vi "AIT 1553 Channel Page.vi"(8 "error in (no error)":errorcluster, 11 "Node Ptr":T1 format="%.0x") -> (0 "error out":errorcluster)   [LabVIEW 2013]
uses:
  <vilib>/NI Veristand/Custom Device API/Custom Device Item Ref.ctl
  Controls and Global/Global.vi
  <vilib>/NI Veristand/Custom Device API/Get Item Property (U32).vi
  <vilib>/NI Veristand/Custom Device API/Set Item Property (U32).vi
  <vilib>/NI Veristand/Custom Device API/Custom Device API.lvlib
  AIT 664 Custom Device.lvlib
panel:
  in  "Input Label Buffer Size":u32
  out "Channel #":u32
  in  "Header":cluster{"Section Name":string}={"Section Name"="AIT 1553 Channel"}
  in  "Description":string
  out "Name":string
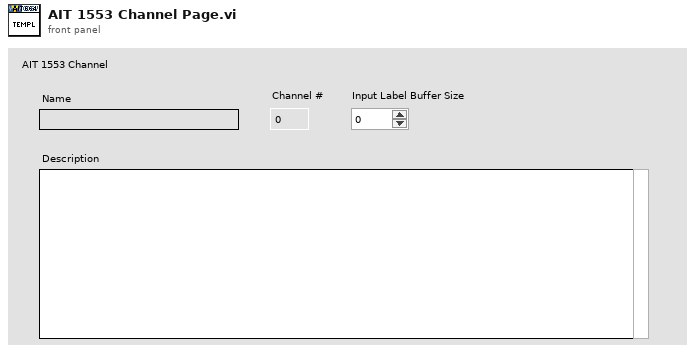
[diagram p1: front panel]
types:
  T1 = typedef "Custom Device API.lvlib/Custom Device Item Ref.ctl" = u64
  T2 = typedef "Custom Device API.lvlib/Custom Device Item Info.ctl" = cluster{"Name":string, "Is Channel":bool, "GUID":string, "Is Waveform":bool}
  T3 = typedef "Custom Device API.lvlib/Custom Device Commands.ctl" = enum16{"Default", "Item renamed", "Shutdown", "Dynamic button pressed"}
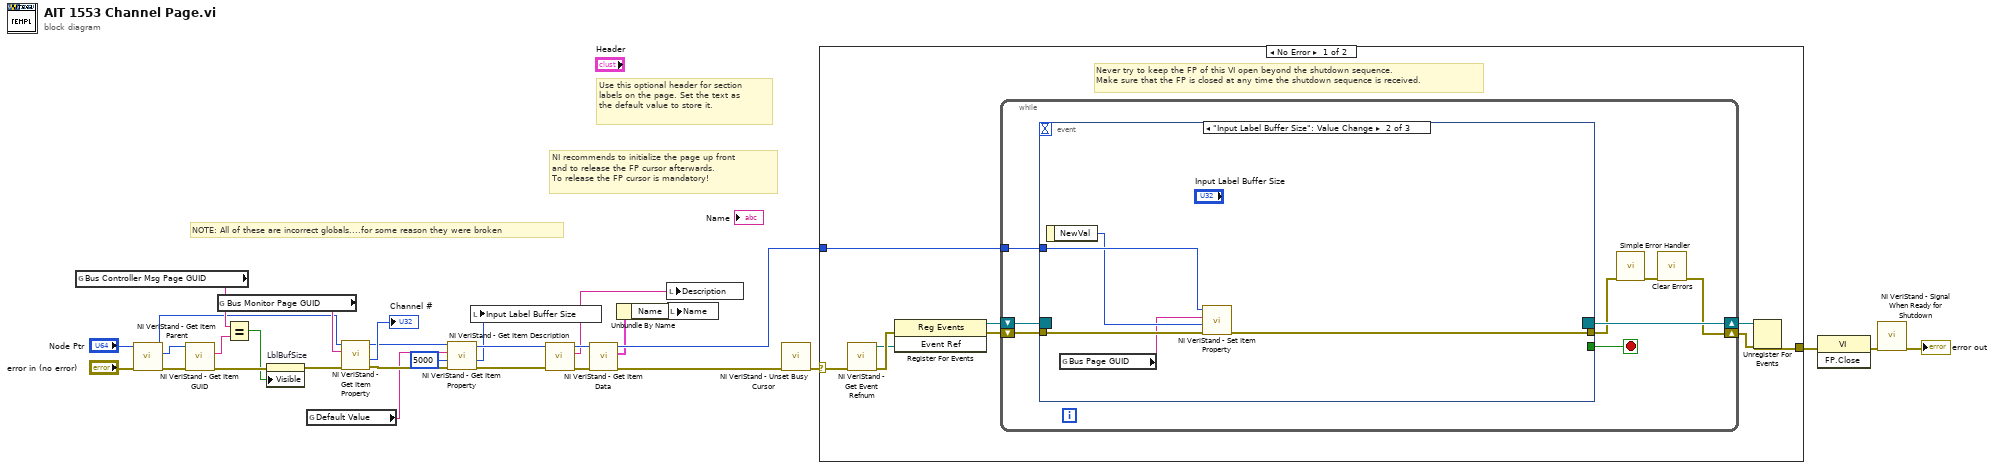
[diagram p0: block diagram]
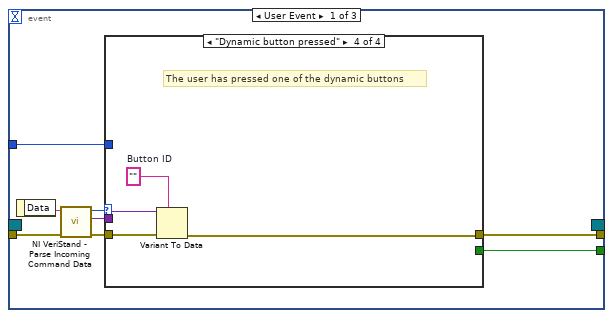
[diagram p2: hidden frame]
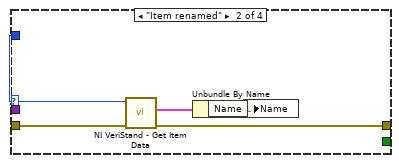
[diagram p4: hidden frame]
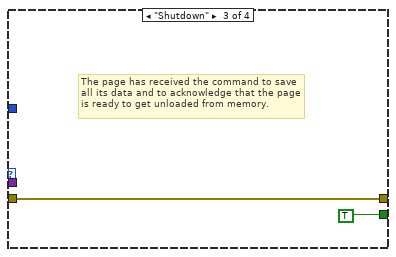
[diagram p5: hidden frame]
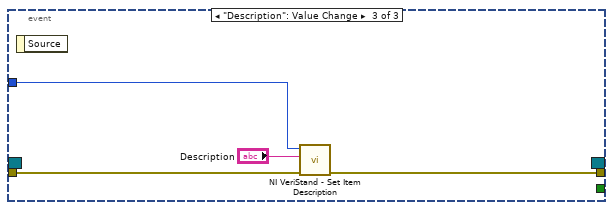
[diagram p6: hidden frame]
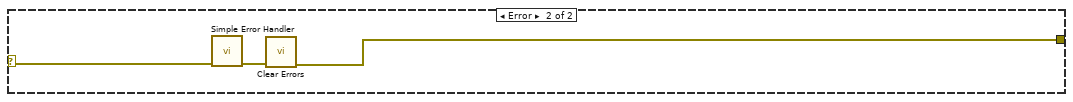
[diagram p7: hidden frame]
diagram:
  # "NOTE: All of these are incorrect globals....for some reason they were broken"
  # "Use this optional header for section labels on the page. Set the text as the default value to store it."
  # "NI recommends to initialize the page up front\nand to release the FP cursor afterwards.\nTo release the FP cursor is mandatory!"
  n1 = global read "Global.vi" "Bus Controller Msg Page GUID"() -> (w9:string)
  n2 = call <vilib>:"NI VeriStand - Get Item Parent.vi"("error in (no error)"="error in (no error)", "Item Ref in"="Node Ptr") -> ("error out"=w4:errorcluster, "Parent Ref"=w5:T1, "Item Ref out"=w6:T1)  [unwired: 6 in, 1 out]
  n3 = call <vilib>:"NI VeriStand - Get Item GUID.vi"("error in (no error)"=w4, "Item Ref in"=w5) -> ("error out"=w3:errorcluster, "GUID"=w10:string)  [unwired: 7 in, 1 out]
  n4 = global read "Global.vi" "Bus Monitor Page GUID"() -> (w19:string)
  n5 = Equal?(x=w9, y=w10) -> (x = y?=w1:bool)
  n6 = property on="LblBufSize" class="DigNum (strict)"(error in=w3, "Visible"=w1) -> (error out=w2:errorcluster)  [unwired: 1 in, 1 out]
  n7 = global read "Global.vi" "Default Value"() -> (w15:string)
  n8 = call-poly <vilib>:"NI VeriStand - Get Item Property.vi"("error in (no error)"=w2, "Property Name"=w19, "Item Ref in"=w6) -> ("error out"=w17:errorcluster, "Value"=→"Channel #":u32, "Item Ref out"=w16:T1)  [unwired: 5 in, 1 out]
  n9 = call-poly <vilib>:"NI VeriStand - Get Item Property.vi"("error in (no error)"=w17, "Default Value"=u32 5000, "Property Name"=w15, "Item Ref in"=w16) -> ("error out"=w13:errorcluster, "Value"=w11:u32, "Item Ref out"=w12:T1)  [unwired: 4 in, 1 out]
  n10 = local write "Input Label Buffer Size"(w11) -> ()
  n11 = call <vilib>:"NI VeriStand - Get Item Description.vi"("error in (no error)"=w13, "Item Ref in"=w12) -> ("error out"=w22:errorcluster, "Description"=w23:string, "Item Ref out"=w24:T1)  [unwired: 7 out]
  n12 = call <vilib>:"NI VeriStand - Get Item Data.vi"("error in (no error)"=w22, "Item Ref in"=w24) -> ("error out"=w27:errorcluster, "Item Info"=w21:T2, "Item Ref out"=w25:T1)  [unwired: 7 out]
  n13 = Unbundle By Name(w21) -> ("Name"=w20:string)
  n14 = local write "Description"(w23) -> ()
  n15 = local write "Name"(w20) -> ()
  n16 = call <vilib>:"NI VeriStand - Unset Busy Cursor.vi"("error in (no error)"=w27) -> ("error out"=w26:errorcluster)  [unwired: 10 out]
  n17 = case shown="No Error" w26 {
    selector: w26 -> [w31 w79]
    tunnel: [w36 w77] -> w30
    tunnel: w25 -> [w32 _]
    frame No Error {
      # "Never try to keep the FP of this VI open beyond the shutdown sequence.\nMake sure that the FP is closed at any time the shutdown sequence is received."
      n18 = call <vilib>:"NI VeriStand - Get Event Refnum.vi"("error in (no error)"=w31) -> ("error out"=w39:errorcluster, "Event Ref"=w35:refnum<user-event>)  [unwired: 9 out]
      n19 = register-events(error in=w39, w35) -> (reference out=w33:refnum<event-registration>, error out=w34:errorcluster)  [unwired: 1 in]
      n20 = while {
        tunnel: w32 -> [w43]
        shift-right: [w40] -> w37
        shift-left: w34 -> [w46]
        shift-right: [w47] -> w38
        shift-left: w33 -> [w45]
        stop <- w44 stop-if-true
        n21 = event shown="[1] \"Input Label Buffer Size\": Value Change" {
          selector: w45 -> [_ _ _]
          dyn-events: [_ _ _] -> w47
          timeout: _ -> [_ _ _]
          tunnel: w46 -> [w55 w72 w75]
          tunnel: [w51 _ _] -> w44
          tunnel: [w50 w68 w74] -> w42
          tunnel: w43 -> [w49 w71 w76]
          event User Event {
            n22 = event-data() -> ("Data"=w54:string)  [unwired: 1 out]
            n23 = call <vilib>:"NI VeriStand - Parse Incoming Command Data.vi"("error in (no error)"=w55, "Incoming data"=w54) -> ("error out"=w53:errorcluster, "Outgoing data"=w48:variant, "Action"=w52:T3)  [unwired: 7 out]
            n24 = case shown="\"Dynamic button pressed\"" w52 {
              tunnel: w53 -> [w56 w61 w62 w67]
              tunnel: [_ _ TRUE _] -> w51
              tunnel: [w56 w58 w62 w64] -> w50
              tunnel: w49 -> [_ w60 _ _]
              tunnel: w48 -> [_ _ _ w66]
              frame "Default", Default {
              }
              frame "Item renamed" {
                n25 = call <vilib>:"NI VeriStand - Get Item Data.vi"("error in (no error)"=w61, "Item Ref in"=w60) -> ("error out"=w58:errorcluster, "Item Info"=w59:T2)  [unwired: 8 out]
                n26 = Unbundle By Name(w59) -> ("Name"=w57:string)
                n27 = local write "Name"(w57) -> ()
              }
              frame "Shutdown" {
                # "The page has received the command to save all its data and to acknowledge that the page is ready to get unloaded from memory."
              }
              frame "Dynamic button pressed" {
                w65 = ""  # Button ID
                # "The user has pressed one of the dynamic buttons"
                n28 = Variant To Data(error in=w67, type=w65, Variant=w66) -> (error out=w64:errorcluster)  [unwired: 1 out]
              }
            }
          }
          event "Input Label Buffer Size": Value Change {
            n29 = event-data() -> ("NewVal"=w70:u32)  [unwired: 1 out]
            n30 = global read "Global.vi" "Bus Page GUID"() -> (w69:string)
            n31 = call-poly <vilib>:"NI VeriStand - Set Item Property.vi"("error in (no error)"=w72, "Value"=w70, "Property Name"=w69, "Item Ref in"=w71) -> ("error out"=w68:errorcluster)  [unwired: 5 in, 2 out]
          }
          event "Description": Value Change {
            n32 = event-data() -> ()  [unwired: 2 out]
            n33 = call <vilib>:"NI VeriStand - Set Item Description.vi"("error in (no error)"=w75, "Description"="Description", "Item Ref in"=w76) -> ("error out"=w74:errorcluster)  [unwired: 8 out]
          }
        }
        n34 = call <vilib>:"Simple Error Handler.vi"("error in (no error)"=w42) -> ("error out"=w41:errorcluster)  [unwired: 1 in, 7 out]
        n35 = call <vilib>:"Clear Errors.vi"("error in (no error)"=w41) -> ("error out"=w40:errorcluster)  [unwired: 6 out]
      }
      n36 = Unregister For Events(event registration refnum=w38, error in=w37) -> (error out=w36:errorcluster)
    }
    frame Error {
      n37 = call <vilib>:"Simple Error Handler.vi"("error in (no error)"=w79) -> ("error out"=w78:errorcluster)  [unwired: 1 in, 7 out]
      n38 = call <vilib>:"Clear Errors.vi"("error in (no error)"=w78) -> ("error out"=w77:errorcluster)  [unwired: 6 out]
    }
  }
  n39 = invoke class="VI" method="FP.Close"(error in=w30) -> (error out=w29:errorcluster)  [unwired: 2 in, 2 out]
  n40 = call <vilib>:"NI VeriStand - Signal When Ready for Shutdown.vi"("error in (no error)"=w29) -> ("error out"=→"error out":errorcluster)  [unwired: 10 out]
